vi "Reference Rectangle.vi"(8 "error in (no error)":errorcluster, 10 "My VI":string, 11 "Ref Top Level in":refnum<class "Ref Top Level.lvclass">) -> (0 "error out":errorcluster, 2 "Rectangle":T1)   [LabVIEW 2017, in "MGI-Panel Manager.lvlib" / "Ref Top Level.lvclass"]
doc: "Returns the center point to use as a reference when positioning the window.\n\n----\nPlease see the following web address for additional documentation and tutorial information:\nhttp://www.mooregoodideas.com/mgi-panel-manager/\n\nAuthor: Derek Trepanier\n\nCopyright (c) 2018, Moore Good Ideas, Inc.\n\nAll rights reserved.\n\nRedistribution and use in source and binary forms, with or without modification, are permitted provided that the following conditions are met:\n\n * Redistributions of source code must retain the above copyright notice, this list of conditions and the following disclaimer.\n * Redistributions in binary form must reproduce the above copyright notice, this list of conditions and the following disclaimer in the documentation and/or other materials provided with the distribution.\n * Neither the name of Moore Good Ideas, Inc. nor the names of its contributors may be used to endorse or promote products derived from this software without specific prior written permission.\n\nTHIS SOFTWARE IS PROVIDED BY THE COPYRIGHT HOLDERS AND CONTRIBUTORS \"AS IS\" AND ANY EXPRESS OR IMPLIED WARRANTIES, INCLUDING, BUT NOT LIMITED TO, THE IMPLIED WARRANTIES OF MERCHANTABILITY AND FITNESS FOR A PARTICULAR PURPOSE ARE DISCLAIMED. IN NO EVENT SHALL THE COPYRIGHT OWNER OR CONTRIBUTORS BE LIABLE FOR ANY DIRECT, INDIRECT, INCIDENTAL, SPECIAL, EXEMPLARY, OR CONSEQUENTIAL DAMAGES (INCLUDING, BUT NOT LIMITED TO, PROCUREMENT OF SUBSTITUTE GOODS OR SERVICES; LOSS OF USE, DATA, OR PROFITS; OR BUSINESS INTERRUPTION) HOWEVER CAUSED AND ON ANY THEORY OF LIABILITY, WHETHER IN CONTRACT, STRICT LIABILITY, OR TORT (INCLUDING NEGLIGENCE OR OTHERWISE) ARISING IN ANY WAY OUT OF THE USE OF THIS SOFTWARE, EVEN IF ADVISED OF THE POSSIBILITY OF SUCH DAMAGE."
uses:
  Ref Top Level.lvclass
  Panel/Panel.lvclass
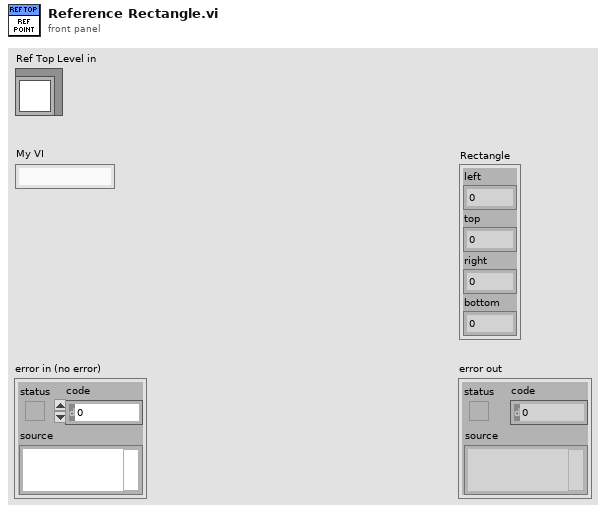
[diagram p1: front panel]
types:
  T1 = cluster{"left":i16, "top":i16, "right":i16, "bottom":i16}
  T2 = enum32{"Invalid", "Standard", "Closed", "Hidden", "Minimized", "Maximized"}[]
  T3 = typedef "LVRectTypeDef.ctl" = cluster{"Left":i16, "Top":i16, "Right":i16, "Bottom":i16}
  T4 = enum32{"Invalid", "Standard", "Closed", "Hidden", "Minimized", "Maximized"}
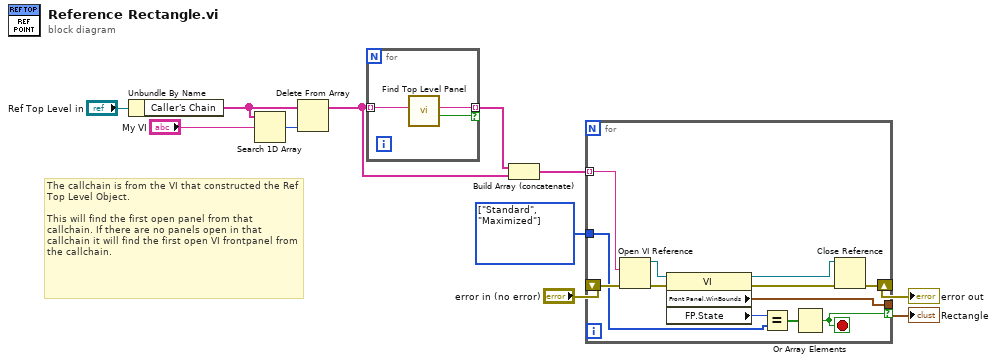
[diagram p0: block diagram]
diagram:
  w7 = T2 [enum."Standard", enum."Maximized"] items=["Invalid", "Standard", "Closed", "Hidden", "Minimized", "Maximized"]
  # "The callchain is from the VI that constructed the Ref Top Level Object.\n\nThis will find the first open panel from that callchain. If there are no panels open in that callchain it will find the first open VI frontpanel from the callchain."
  n1 = Unbundle By Name("Ref Top Level in") -> ("Caller's Chain"=w6:string[])
  n2 = Search 1D Array(1D array=w6, element="My VI") -> (index of element=w5:i32)  [unwired: 1 in]
  n3 = Delete From Array(array=w6, index=w5) -> (array with subset deleted=w2:string[])  [unwired: 1 in, 1 out]
  n4 = for {
    tunnel: w2 -> [w14] mode=indexing
    tunnel: [w13] -> w3 mode=indexing if=w12
    n5 = call "Find Top Level Panel.vi"("VI (Caller)"=w14) -> ("Found?"=w12:bool, "Top Level Panel"=w13:string)  [unwired: 9 in]
  }
  n6 = Build Array (concatenate)(w3, w2) -> (w1:string[])
  n7 = for {
    tunnel: [w26] -> w11 if=w16
    shift-right: [w20] -> w9
    shift-left: "error in (no error)" -> [w25]
    tunnel: w7 -> [w18]
    tunnel: w1 -> [w15] mode=indexing
    stop <- w16 stop-if-true
    n8 = Open VI Reference(vi path=w15, error in (no error)=w25) -> (vi reference=w23:refnum<vi>, error out=w24:errorcluster)  [unwired: 4 in]
    n9 = property class="VI"(reference=w23, error in=w24) -> (reference out=w22:refnum<vi>, error out=w21:errorcluster, "Front Panel.WinBounds"=w26:T3, "FP.State"=w19:T4)
    n10 = Equal?(x=w19, y=w18) -> (x = y?=w17:bool[])
    n11 = Or Array Elements(Boolean array=w17) -> (logical OR=w16:bool)
    n12 = Close Reference(reference=w22, error in (no error)=w21) -> (error out=w20:errorcluster)
  }
  "error out" <- w9
  "Rectangle" <- w11
